vi "Example Read File - Allocate String.vi"(8 "buffer":string, 9 "session id":i32, 10 "error in":errorcluster, 11 "reference in":refnum<k24>) -> (1 "string id":i32, 2 "error out":errorcluster, 3 "reference out":refnum<k24>)   [LabVIEW 2010]
uses:
  C:/tf/play/labview/Tinkerforge.dll
  Tinkerforge.dll
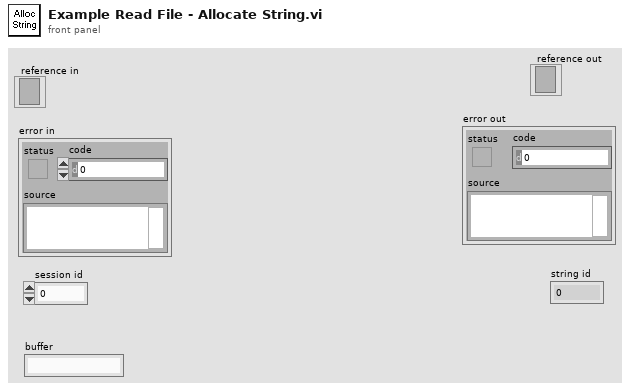
[diagram p1: front panel]
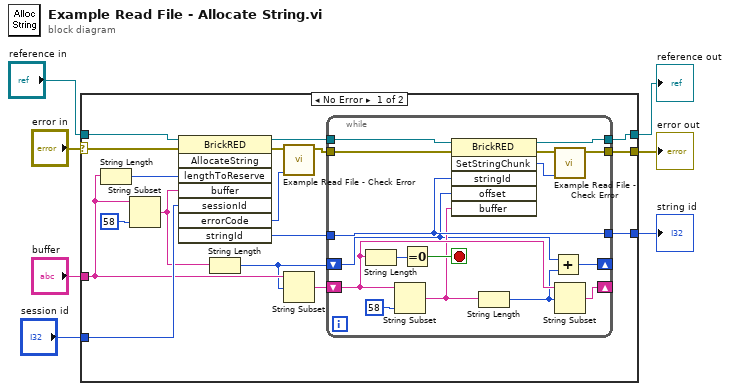
[diagram p0: block diagram]
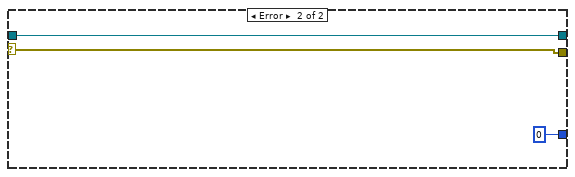
[diagram p2: hidden frame]
diagram:
  n1 = case shown="No Error" "error in" {
    selector: "error in" -> [w24 w43]
    tunnel: [w15 w43] -> w6
    tunnel: [w16 w42] -> w5
    tunnel: "reference in" -> [w23 w42]
    tunnel: "session id" -> [w20 _]
    tunnel: "buffer" -> [w12 _]
    tunnel: [w13 0 ("stringId")] -> w1
    frame No Error {
      n2 = String Length(string=w12) -> (length=w19:i32)
      n3 = String Subset(string=w12, length (rest)=58 ("length (rest)")) -> (substring=w9:string)  [unwired: 1 in]
      n4 = invoke class="BrickRED" method="AllocateString"(reference=w23, error in=w24, "lengthToReserve"=w19, "buffer"=w9, "sessionId"=w20) -> (reference out=w17:refnum<k24>, error out=w22:errorcluster, "errorCode"=w21:u8, "stringId"=w14:i32)  [unwired: 3 in, 4 out]
      n5 = String Length(string=w9) -> (length=w8:i32)
      n6 = call "Example Read File - Check Error.vi"("error code"=w21, "error in"=w22) -> ("error out"=w18:errorcluster)  [unwired: 9 in]
      n7 = String Subset(string=w12, offset (0)=w8) -> (substring=w10:string)  [unwired: 1 in]
      n8 = while {
        tunnel: w18 -> [w40]
        tunnel: [w31] -> w15
        tunnel: w17 -> [w39]
        tunnel: [w38] -> w16
        tunnel: w14 -> [w37]
        tunnel: [w37] -> w13
        shift-right: [w33] -> _
        shift-left: w10 -> [w29]
        shift-right: [w25] -> _
        shift-left: w8 -> [w27]
        stop <- w35 stop-if-true
        n9 = String Length(string=w29) -> (length=w36:i32)
        n10 = String Subset(string=w29, length (rest)=58) -> (substring=w28:string)  [unwired: 1 in]
        n11 = Equal To 0?(x=w36) -> (x = 0?=w35:bool)
        n12 = invoke class="BrickRED" method="SetStringChunk"(reference=w39, error in=w40, "stringId"=w37, "offset"=w27, "buffer"=w28) -> (reference out=w38:refnum<k24>, error out=w32:errorcluster, "SetStringChunk"=w30:u8)  [unwired: 1 in, 3 out]
        n13 = String Length(string=w28) -> (length=w26:i32)
        n14 = Add(x=w27, y=w26) -> (x+y=w25:i32)
        n15 = call "Example Read File - Check Error.vi"("error code"=w30, "error in"=w32) -> ("error out"=w31:errorcluster)  [unwired: 9 in]
        n16 = String Subset(string=w29, offset (0)=w26) -> (substring=w33:string)  [unwired: 1 in]
      }
    }
    frame Error {
    }
  }
  "error out" <- w6
  "reference out" <- w5
  "string id" <- w1
